vi "Stop Core.vi"(10 "final error code":i32, 11 "UI Wizard in":refnum<class "UI Wizard.lvclass">) -> (3 "UI Wizard out":refnum<class "UI Wizard.lvclass">)   [LabVIEW 2013, in "SET Project Editor.lvlib" / "UI Wizard.lvclass"]
doc: "(<B>Filename</B>: Actor Framework.lvlib:Actor.lvclass:Stop Core.vi)\n\nDefines what the actor does before it stops. Use the <B>final error code</B> input to determine whether the actor shut down in response to an error.\n\nBy default, this method does nothing. A descendant class may override it to define behavior, such as shutting down any processes the actor initiated in its override of the Actor Core method."
uses:
  UI Wizard.lvclass
  UI Actor/UI Actor.lvclass
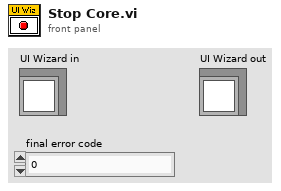
[diagram p1: front panel]
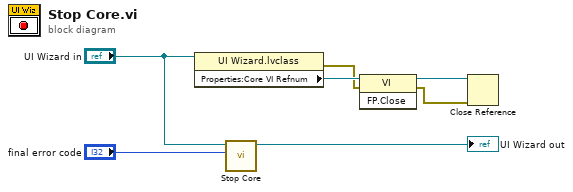
[diagram p0: block diagram]
diagram:
  n1 = property class="UI Wizard.lvclass"(reference="UI Wizard in") -> (error out=w1:errorcluster, "Properties:Core VI Refnum"=w4:refnum<vi>)  [unwired: 1 in, 1 out]
  n2 = call-parent "Stop Core.vi"("final error code"="final error code", "UI Actor in"="UI Wizard in") -> ("UI Actor out"=→"UI Wizard out":refnum<class "UI Wizard.lvclass">)  [unwired: 9 in]
  n3 = invoke class="VI" method="FP.Close"(reference=w4, error in=w1) -> (reference out=w3:refnum<vi>, error out=w2:errorcluster)  [unwired: 1 in, 1 out]
  n4 = Close Reference(reference=w3, error in (no error)=w2) -> ()  [unwired: 1 out]
